vi "setSamplingMode.vi"(8 "error in (no error)":errorcluster, 10 "Fs Mode":T1, 11 "Instrument.LockinAPI in":refnum<class "Instrument.LockinAPI.lvclass">) -> (0 "error out":errorcluster, 3 "Instrument.LockinAPI out":refnum<class "Instrument.LockinAPI.lvclass">)   [LabVIEW 2019, in "Instrument.LockinAPI.lvclass"]
doc: "API to put lockin into IV mode.\n\nIf address=\"\", this API reads from localhost\nIf address is remote lockin, you need to add this computer to allowed whitelist on the lockin computer you are trying to access."
uses:
  Instrument.LockinAPI.lvclass
  Typedefs/API/LockinAPI.Sampling.FsMode--enum.ctl
  Typedefs/API/LockinAPI.Commands--Enum.ctl
  08458c74-1ef2-45d6-87a0-b6580aa97565.vi
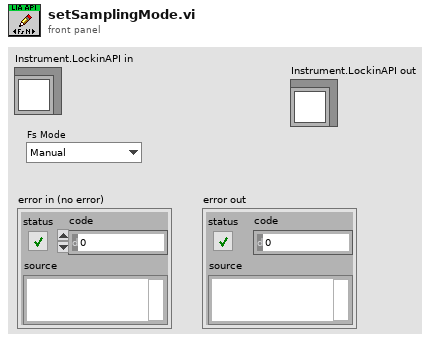
[diagram p1: front panel]
types:
  T1 = typedef "Instrument.LockinAPI.lvclass/LockinAPI.Sampling.FsMode--enum.ctl" = enum16{"Manual", "Auto Fs", "Max Fs"}
  T2 = typedef "Instrument.LockinAPI.lvclass/LockinAPI.Commands--Enum.ctl" = enum16{"setAI", "setAO", "setAO_Amplitude", "setAO_DC", "setAO_Frequency", "setAO_Phase", "setAO_Function", "setAO_I+", "setREF", "setREF_Frequency", "setREF_Phase", "setREF_TC", "setREF_Roll-Off", "setDAQ", "setSampling", "setOffset", "setState", "getState", "getAO", "getAI", "getResults", "getSampling", "getAOconfig", "getREFconfig", "setInputGain", "setOutputGain", "getInputGain", "getOutputGain", "setSamplingMode", "getSamplingMode", "setSweep", "setSweepTime", "setSweepTable", "getStatus", "getSweepResults", "getSweepWaveforms", "startSweep", "stopSweep", "setAUX", "getAUX"}
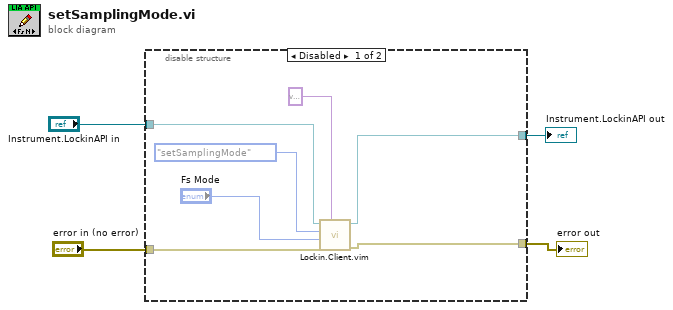
[diagram p0: block diagram]
diagram:
  n1 = disable-structure shown="Disabled" {
    disable-tunnel: [w9 w13] -> w4
    disable-tunnel: [w8 w12] -> w3
    disable-tunnel: "Instrument.LockinAPI in" -> [w6 w13]
    disable-tunnel: "error in (no error)" -> [w7 w12]
    frame Disabled {
      n2 = call "Lockin.Client.vim"("Data Out type"=variant, "error in (no error)"=w7, "Data"="Fs Mode", "Command"=LockinAPI.Commands--Enum."setSamplingMode", "Instrument.LockinAPI in"=w6) -> ("error out"=w8:errorcluster, "Instrument.LockinAPI out"=w9:refnum<class "Instrument.LockinAPI.lvclass">)  [unwired: 4 in, 1 out]
    }
    frame Enabled {
    }
  }
  "Instrument.LockinAPI out" <- w4
  "error out" <- w3
